vi "NI_Tach_Digital.vi"() -> ()   [LabVIEW 2020]
uses:
  <extravilib>/ChannelInstances/Tag-bool.lvlib
  <vilib>/Utility/error.llb/DialogType.ctl
  <vilib>/Waveform/DWDTOps.llb/DWDT Digital to Binary U32.vi
  <vilib>/Waveform/WDTFileIO.llb/ Write Waveform to File (Digital).vi
  <vilib>/Waveform/WDTFileIO.llb/Export Waveforms To Spreadsheet File (Digital).vi
panel:
  out "Tach Graph 4":digitalwaveform[](graph)
  out "Tach Graph 3":digitalwaveform[](graph)
  out "Tach Graph 2":digitalwaveform[](graph)
  out "Tach Graph":digitalwaveform[](graph)
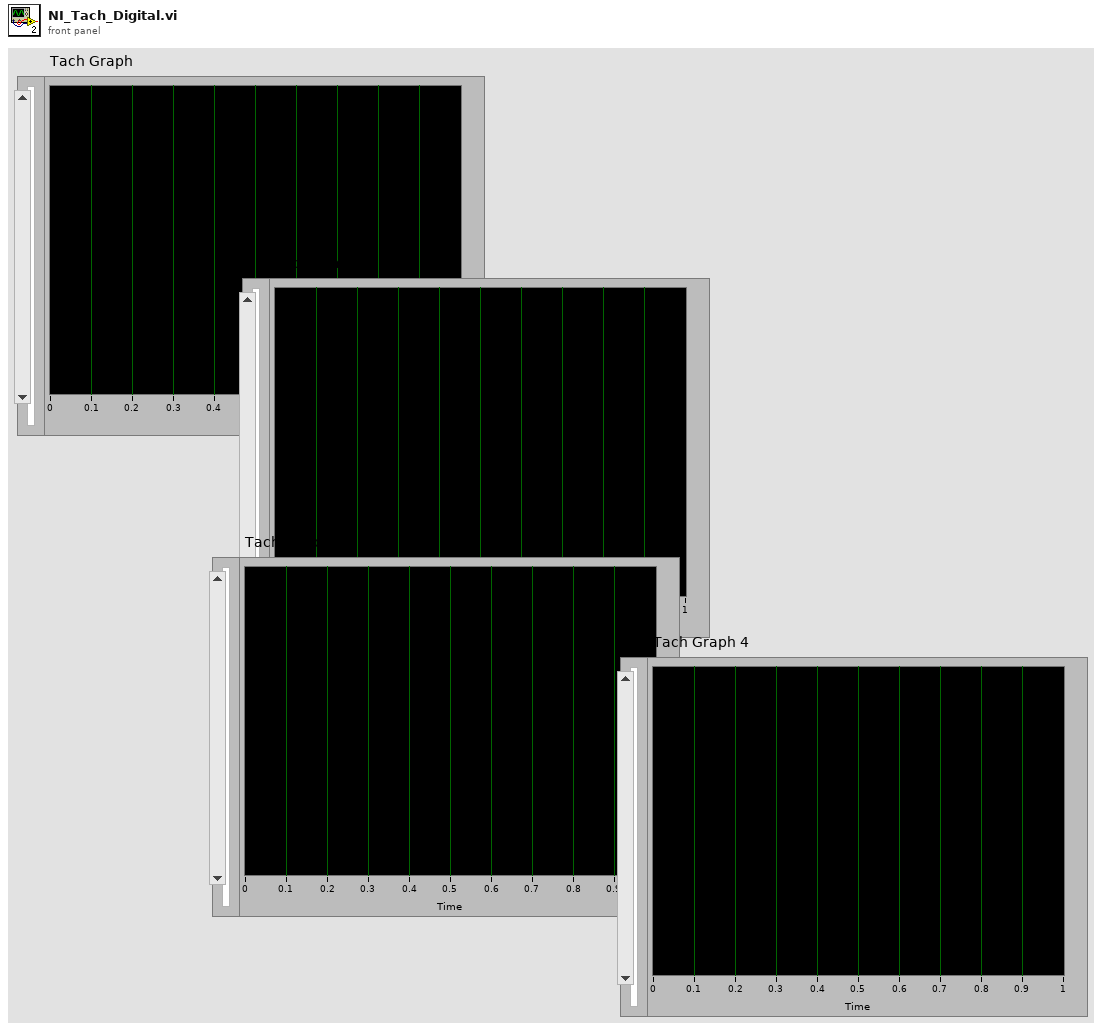
[diagram p1: front panel]
types:
  T1 = typedef "DialogType.ctl" = u16
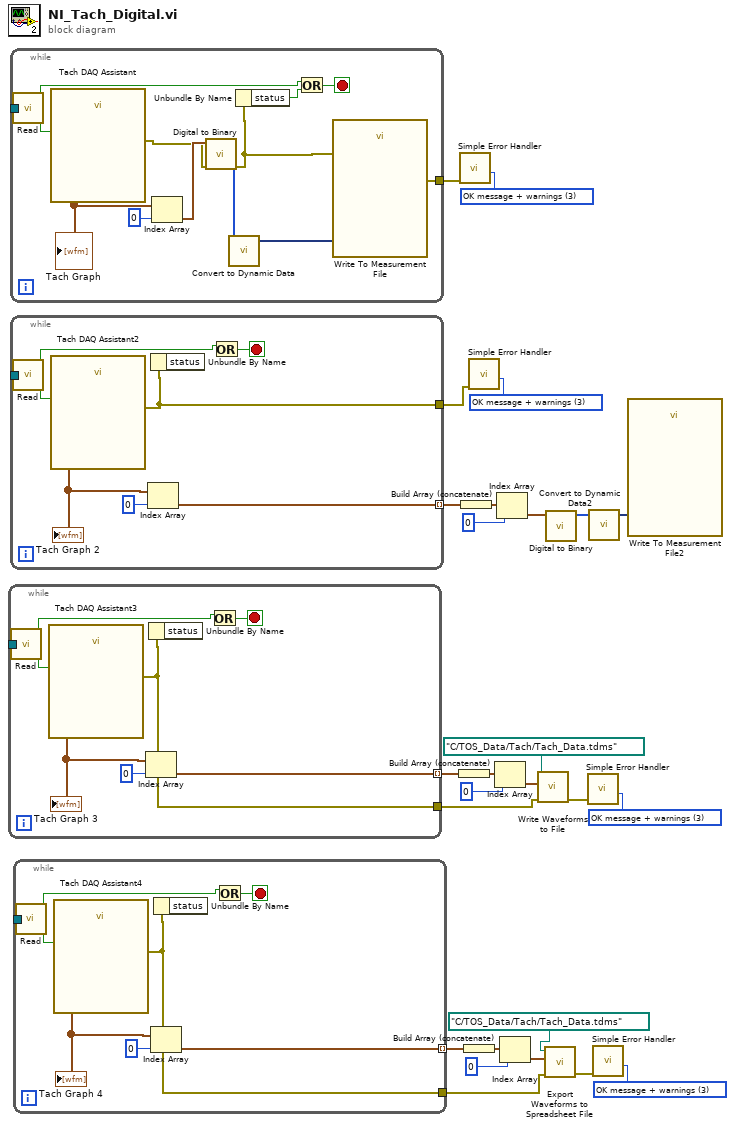
[diagram p0: block diagram]
diagram:
  w2 = T1 3 items=["no dialog", "OK message", "continue or stop message", "OK message + warnings", "continue/stop + warnings"] ("type of dialog (OK msg:1)")
  w11 = T1 3 items=["no dialog", "OK message", "continue or stop message", "OK message + warnings", "continue/stop + warnings"] ("type of dialog (OK msg:1)")
  w24 = T1 3 items=["no dialog", "OK message", "continue or stop message", "OK message + warnings", "continue/stop + warnings"] ("type of dialog (OK msg:1)")
  w26 = T1 3 items=["no dialog", "OK message", "continue or stop message", "OK message + warnings", "continue/stop + warnings"] ("type of dialog (OK msg:1)")
  n1 = while {
    tunnel: _ -> [w33]
    tunnel: [w28] -> w8
    tunnel: [w27] -> w16 mode=indexing
    stop <- w32 stop-if-true
    n2 = call <extravilib>:"Read.vi"("channel"=w33) -> ("element"=w31:bool)  [unwired: 1 in, 1 out]
    n3 = call "Tach DAQ Assistant3"("stop (F)"=w31) -> ("data"=w29:digitalwaveform[], "error out"=w28:errorcluster)  [unwired: 15 in, 2 out]
    "Tach Graph 3" <- w29
    n4 = Index Array(array=w29, index=0) -> (element=w27:digitalwaveform)
    n5 = Unbundle By Name(w28) -> ()  [unwired: 1 out]
    n6 = Or(x=w31) -> (x .or. y?=w32:bool)  [unwired: 1 in]
  }
  n7 = while {
    tunnel: _ -> [w45]
    tunnel: [w41] -> w25
    stop <- w44 stop-if-true
    n8 = call <extravilib>:"Read.vi"("channel"=w45) -> ("element"=w42:bool)  [unwired: 1 in, 1 out]
    n9 = call "Tach DAQ Assistant"("stop (F)"=w42) -> ("data"=w38:digitalwaveform[], "error out"=w35:errorcluster)  [unwired: 15 in, 2 out]
    "Tach Graph" <- w38
    n10 = Index Array(array=w38, index=0) -> (element=w36:digitalwaveform)
    n11 = call-poly <vilib>:"Digital to Binary.vi"("error in (no error)"=w35, "digital waveform"=w36) -> ("error out"=w34:errorcluster, "binary array"=w40:u32[])  [unwired: 8 in]
    n12 = call "Convert to Dynamic Data"("Array"=w40) -> ("Dynamic Data Type"=w39:dynamicdata)  [unwired: 3 in]
    n13 = Unbundle By Name(w34) -> ("status"=w43:bool)
    n14 = Or(x=w42, y=w43) -> (x .or. y?=w44:bool)
    n15 = call "Write To Measurement File"("Signals"=w39, "error in (no error)"=w34) -> ("error out"=w41:errorcluster)  [unwired: 15 in, 2 out]
  }
  n16 = while {
    tunnel: _ -> [w52]
    tunnel: [w47] -> w23
    tunnel: [w46] -> w22 mode=indexing
    stop <- w51 stop-if-true
    n17 = call <extravilib>:"Read.vi"("channel"=w52) -> ("element"=w50:bool)  [unwired: 1 in, 1 out]
    n18 = call "Tach DAQ Assistant2"("stop (F)"=w50) -> ("data"=w48:digitalwaveform[], "error out"=w47:errorcluster)  [unwired: 15 in, 2 out]
    "Tach Graph 2" <- w48
    n19 = Index Array(array=w48, index=0) -> (element=w46:digitalwaveform)
    n20 = Unbundle By Name(w47) -> ()  [unwired: 1 out]
    n21 = Or(x=w50) -> (x .or. y?=w51:bool)  [unwired: 1 in]
  }
  n22 = while {
    tunnel: _ -> [w59]
    tunnel: [w54] -> w4
    tunnel: [w53] -> w6 mode=indexing
    stop <- w58 stop-if-true
    n23 = call <extravilib>:"Read.vi"("channel"=w59) -> ("element"=w57:bool)  [unwired: 1 in, 1 out]
    n24 = call "Tach DAQ Assistant4"("stop (F)"=w57) -> ("data"=w55:digitalwaveform[], "error out"=w54:errorcluster)  [unwired: 15 in, 2 out]
    "Tach Graph 4" <- w55
    n25 = Index Array(array=w55, index=0) -> (element=w53:digitalwaveform)
    n26 = Unbundle By Name(w54) -> ()  [unwired: 1 out]
    n27 = Or(x=w57) -> (x .or. y?=w58:bool)  [unwired: 1 in]
  }
  n28 = Build Array (concatenate)(w16) -> (w15:digitalwaveform[])
  n29 = call <vilib>:"Simple Error Handler.vi"("type of dialog (OK msg:1)"=w26, "error in (no error)"=w25) -> ()  [unwired: 3 in, 5 out]
  n30 = Build Array (concatenate)(w22) -> (w21:digitalwaveform[])
  n31 = Build Array (concatenate)(w6) -> (w10:digitalwaveform[])
  n32 = call <vilib>:"Simple Error Handler.vi"("type of dialog (OK msg:1)"=w24, "error in (no error)"=w23) -> ()  [unwired: 3 in, 5 out]
  n33 = Index Array(array=w15, index=0) -> (element=w13:digitalwaveform)
  n34 = Index Array(array=w21, index=0) -> (element=w19:digitalwaveform)
  n35 = Index Array(array=w10, index=0) -> (element=w5:digitalwaveform)
  n36 = call-poly <vilib>:"Write Waveforms to File.vi"("error in (no error)"=w8, "waveform"=w13, "file path (dialog if empty)"=path "C:/TOS_Data/Tach/Tach_Data.tdms") -> ("error out"=w7:errorcluster)  [unwired: 7 in, 1 out]
  n37 = call-poly <vilib>:"Export Waveforms to Spreadsheet File.vi"("error in (no error)"=w4, "Digital Waveform"=w5, "file path (dialog if empty)"=path "C:/TOS_Data/Tach/Tach_Data.tdms") -> ("error out"=w1:errorcluster)  [unwired: 7 in, 1 out]
  n38 = call-poly <vilib>:"Digital to Binary.vi"("digital waveform"=w19) -> ("binary array"=w18:u32[])  [unwired: 9 in, 1 out]
  n39 = call <vilib>:"Simple Error Handler.vi"("type of dialog (OK msg:1)"=w11, "error in (no error)"=w7) -> ()  [unwired: 3 in, 5 out]
  n40 = call "Convert to Dynamic Data2"("Array"=w18) -> ("Dynamic Data Type"=w17:dynamicdata)  [unwired: 3 in]
  n41 = call <vilib>:"Simple Error Handler.vi"("type of dialog (OK msg:1)"=w2, "error in (no error)"=w1) -> ()  [unwired: 3 in, 5 out]
  n42 = call "Write To Measurement File2"("Signals"=w17) -> ()  [unwired: 16 in, 3 out]
